vi "Init PWM.vi"(7 "Phase-Correct (F)":bool, 8 "error in (no error)":errorcluster, 9 "Enable (F)":bool, 10 "Channel":i32, 11 "VISA resource name in":refnum<visa-resource-name>) -> (0 "error out":errorcluster, 3 "VISA resource name":refnum<visa-resource-name>)   [LabVIEW 2020, in "CTI-Visa.lvlib"]
uses:
  CTI-Visa.lvlib
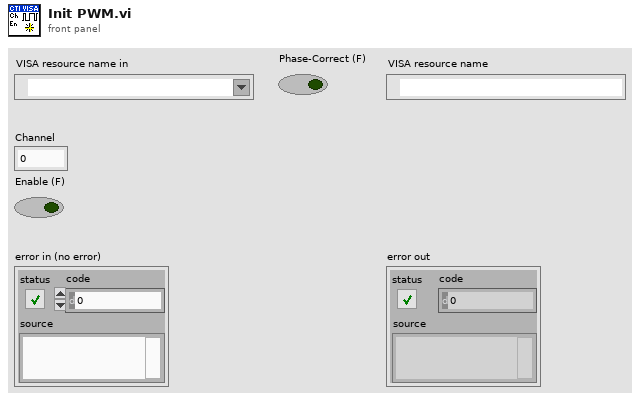
[diagram p1: front panel]
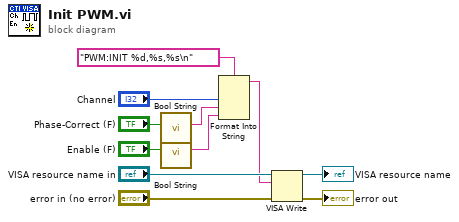
[diagram p0: block diagram]
diagram:
  n1 = call "Bool String.vi"("Bool"="Phase-Correct (F)") -> ("String"=w8:string)  [unwired: 10 in]
  n2 = call "Bool String.vi"("Bool"="Enable (F)") -> ("String"=w7:string)  [unwired: 10 in]
  n3 = Format Into String(format string="PWM:INIT %d,%s,%s\n", "Channel", w8, w7) -> (resulting string=w1:string)  [unwired: 2 in, 1 out]
  n4 = VISA Write(VISA resource name="VISA resource name in", write buffer=w1, error in (no error)="error in (no error)") -> (VISA resource name out=→"VISA resource name":refnum<visa-resource-name>, error out=→"error out":errorcluster)  [unwired: 1 out]
